vi "dfd_Get Alternate Components of Array (Real).vi"(11 "input array":i32[](array[numeric])) -> (2 "another half":i32[](array[numeric]), 3 "half array":i32[](array[numeric]))   [LabVIEW 2017, in "NI_DigFilterLicensed.lvlib"]
uses:
  <vilib>/addons/Digital Filter Design/NI_DigFilterLicensed.lvlib
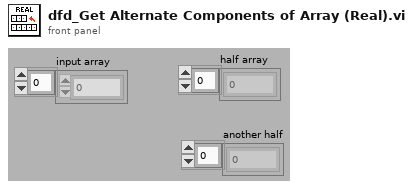
[diagram p1: front panel]
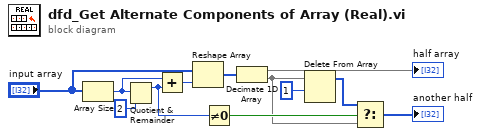
[diagram p0: block diagram]
diagram:
  n1 = Array Size(array="input array") -> (size(s)=w8:i32)
  n2 = Quotient & Remainder(x=w8, y=2) -> (x-y*floor(x/y)=w6:i32)  [unwired: 1 out]
  n3 = Add(x=w8, y=w6) -> (x+y=w9:i32)
  n4 = Reshape Array("input array", w9) -> (w7:i32[])
  n5 = Not Equal To 0?(x=w6) -> (x != 0?=w4:bool)
  n6 = Decimate 1D Array(w7) -> (→"half array":i32[], w2:i32[])
  n7 = Delete From Array(array=w2, length=1) -> (array with subset deleted=w3:i32[])  [unwired: 1 in, 1 out]
  n8 = Select(t=w3, s=w4, f=w2) -> (s? t:f=→"another half":i32[])
